vi "Initialize AO Task.vi"(8 "error in (no error)":errorcluster, 11 "BNT_ULx-MCSV in":refnum<class "BNT_ULx-MCSV.lvclass">) -> (0 "error out":errorcluster, 3 "AO ULx Task":refnum<k24>)   [LabVIEW 2020, in "BNT_ULx.lvlib" / "BNT_ULx-MCSV.lvclass"]
doc: "Initialize ULx Analog Output task.\n\n<b>Default Implementation:</b> Analog Output Voltage\n\nThis dynamic dispatch VI can be overritten by derived classes to implement other analog output tasks."
uses:
  BNT_ULx-MCSV.lvclass
  C:/Program Files (x86)/National Instruments/LabVIEW 2020/vi.lib/ULx/ULx_LV.dll
  Program Files (x86)/National Instruments/LabVIEW 2020/vi.lib/ULx/ULx_LV.dll
  BNT_ULx-MCSV.lvclass/BNT_ULx-MCSV.ctl
  <vilib>/ULx/Create Channel.llb/ULx Create Channel (AO-Voltage-Basic).vi
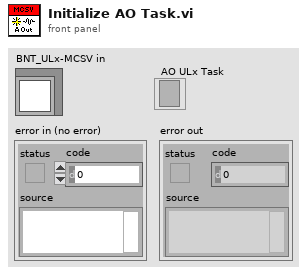
[diagram p1: front panel]
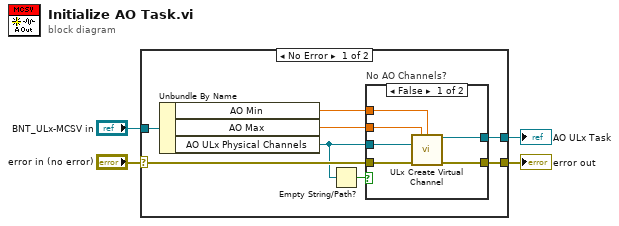
[diagram p0: block diagram]
diagram:
  n1 = case shown="No Error" "error in (no error)" {
    selector: "error in (no error)" -> [w8 w20]
    tunnel: [w12 w20] -> w3
    tunnel: "BNT_ULx-MCSV in" -> [w5 _]
    tunnel: [w11 _] -> w1
    frame No Error {
      n2 = Unbundle By Name(w5) -> ("AO Min"=w10:dbl, "AO Max"=w9:dbl, "AO ULx Physical Channels"=w6:refnum<k21>)
      n3 = Empty String/Path?(string/path=w6) -> (empty?=w7:bool)
      n4 = case "No AO Channels?" shown="False" w7 {
        tunnel: w6 -> [w16 _]
        tunnel: [w17 w19] -> w12
        tunnel: [w13 _] -> w11
        tunnel: w10 -> [w15 _]
        tunnel: w9 -> [w14 _]
        tunnel: w8 -> [w18 w19]
        frame False {
          n5 = call-poly <vilib>:"ULx Create Virtual Channel.vi"("maximum value"=w14, "minimum value"=w15, "physical channels"=w16, "error in"=w18) -> ("task out"=w13:refnum<k24>, "error out"=w17:errorcluster)  [unwired: 10 in]
        }
        frame True {
        }
      }
    }
    frame Error {
    }
  }
  "error out" <- w3
  "AO ULx Task" <- w1
